vi "Traffic_Light.vi"() -> ()   [LabVIEW 2024]
panel:
  out "Boolean 3":bool
  out "Boolean 2":bool
  out "Boolean":bool
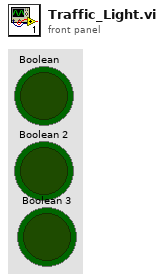
[diagram p1: front panel]
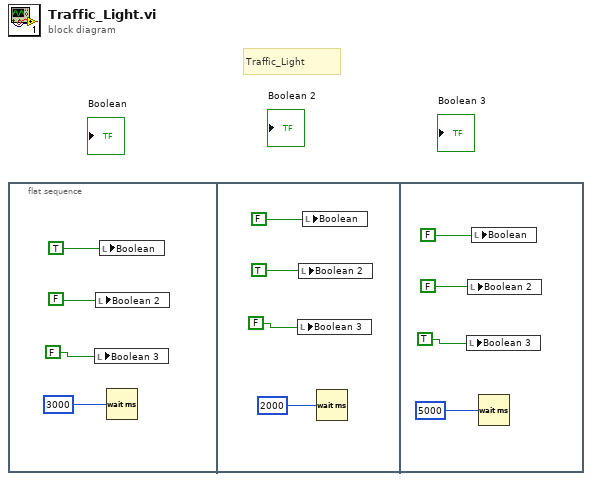
[diagram p0: block diagram]
diagram:
  # "Traffic_Light"
  n1 = flat-sequence {
    frame #0 {
      n2 = local write "Boolean 3"(FALSE) -> ()
      n3 = local write "Boolean 2"(FALSE) -> ()
      n4 = local write "Boolean"(TRUE) -> ()
      n5 = Wait (ms)(milliseconds to wait=3000) -> ()  [unwired: 1 out]
    }
    frame #1 {
      n6 = local write "Boolean 3"(FALSE) -> ()
      n7 = local write "Boolean 2"(TRUE) -> ()
      n8 = local write "Boolean"(FALSE) -> ()
      n9 = Wait (ms)(milliseconds to wait=2000) -> ()  [unwired: 1 out]
    }
    frame #2 {
      n10 = local write "Boolean 3"(TRUE) -> ()
      n11 = local write "Boolean 2"(FALSE) -> ()
      n12 = local write "Boolean"(FALSE) -> ()
      n13 = Wait (ms)(milliseconds to wait=5000) -> ()  [unwired: 1 out]
    }
  }
